vi "InitActuators.vi"   [LabVIEW 2020]
doc: "This VI initializes miscellaneous devices such as the compressor and any decorations."
uses:
  <vilib>/Rock Robotics/WPI/Utilities/WPI_GetSetVariantRefNum.vi
  <vilib>/Rock Robotics/WPI/ThirdParty/Phoenix-LabVIEW/Motor Controller/Controls/CTRE_Phoenix_MotorControl_TalonFXInvertType.ctl
  <vilib>/Rock Robotics/WPI/ThirdParty/Phoenix-LabVIEW/Motor Controller/Controls/CTRE_Phoenix_MotorControl_NeutralMode.ctl
  <vilib>/Rock Robotics/WPI/ThirdParty/Phoenix-LabVIEW/Motor Controller/Controls/CTRE_Phoenix_MotorControl_FeedbackDevice_TalonFX.ctl
  <vilib>/Rock Robotics/WPI/ThirdParty/Phoenix-LabVIEW/Motor Controller/Controls/CTRE_Phoenix_MotorControl_SupplyCurrentLimitConfiguration.ctl
  <vilib>/Rock Robotics/WPI/ThirdParty/Phoenix-LabVIEW/Motor Controller/Controls/CTRE_Phoenix_MotorControl_StatusFrameEnhanced.ctl
  GlobalActuators.vi
types:
  T1 = typedef "CTRE_Phoenix_MotorControl_StatusFrameEnhanced.ctl" = u16
  T2 = typedef "CTRE_Phoenix_MotorControl_SupplyCurrentLimitConfiguration.ctl" = cluster{"Enable?":bool, "Current Limit":dbl, "Threshold Current":dbl, "Threshold Time":dbl}
  T3 = typedef "CTRE_Phoenix_MotorControl_FeedbackDevice_TalonFX.ctl" = i8
  T4 = typedef "CTRE_Phoenix_MotorControl_NeutralMode.ctl" = enum8{"EEPROMSetting", "Override to Coast", "Override to Brake"}
  T5 = typedef "CTRE_Phoenix_MotorControl_TalonFXInvertType.ctl" = enum16{"Counter-Clockwise", "Clockwise"}
  T6 = typedef "WPI_MotorControlDeviceRef.ctl" = cluster{"DeviceStatus":errorcluster, "Type":T7, "PWM":cluster{"PWM Channel":T8, "DeadBand":T9}, "CAN":cluster{"Device Number":u8, "SetOutput VI Ref":variant, "GetOutput VI Ref":variant, "Enable VI Ref":variant, "Disable VI Ref":variant, "Data":variant}, "Invert":bool, "DIO PWM":cluster{"PWM \"Enable\" Channel":T8, "DIOChannel":T10, "PWM Rate":dbl}}
  T7 = typedef "WPI_MotorControlType.ctl" = enum16{"PWM", "CAN", "DIO PWM"}
  T8 = typedef "FPGA_DIOPWMChannel.ctl" = enum8{"PWM 0", "PWM 1", "PWM 2", "PWM 3", "PWM 4", "PWM 5", "PWM 6", "PWM 7", "PWM 8", "PWM 9", "PWM MXP 0", "PWM MXP 1", "PWM MXP 2", "PWM MXP 3", "PWM MXP 4", "PWM MXP 5", "PWM MXP 6", "PWM MXP 7", "PWM MXP 8", "PWM MXP 9", "Invalid"}
  T9 = typedef "WPI_PWMDeadband.ctl" = cluster{"Name":string, "maxPositivePwm":i32, "minPositivePwm":i32, "centerPwm":i32, "maxNegativePwm":i32, "minNegativePwm":i32, "angularRange":u16}
  T10 = typedef "FPGA_DIOChannel.ctl" = enum8{"DIO 0", "DIO 1", "DIO 2", "DIO 3", "DIO 4", "DIO 5", "DIO 6", "DIO 7", "DIO 8", "DIO 9", "DIO MXP 0", "DIO MXP 1", "DIO MXP 2", "DIO MXP 3", "DIO MXP 4", "DIO MXP 5", "DIO MXP 6", "DIO MXP 7", "DIO MXP 8", "DIO MXP 9", "DIO MXP 10", "DIO MXP 11", "DIO MXP 12", "DIO MXP 13", "DIO MXP 14", "DIO MXP 15", "SPI Port CS1", "SPI Port CS2", "SPI Port CS3", "SPI Port MISO", "SPI Port MOSI", "Invalid"}
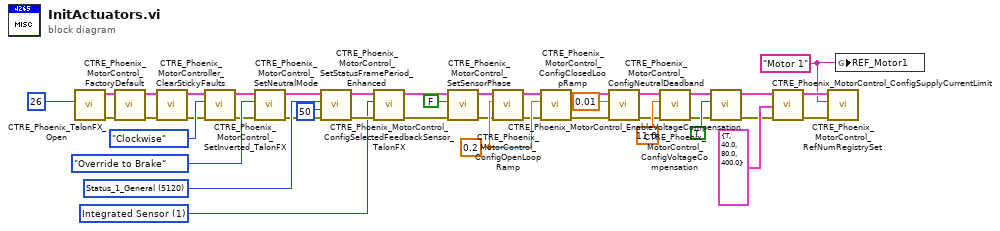
[diagram p0: block diagram]
diagram:
  w25 = T1 5120 items=["Status_1_General"=5120, "Status_2_Feedback0"=5184, "Status_3_Quadrature"=5248, "Status_4_AinTempVbat"=5312, "Status_6_Misc"=5440, "Status_7_CommStatus"=5504, "Status_8_PulseWidth"=5568, "Status_9_MotProfBuffer"=5632, "Status_10_MotionMagic"=5696, "Status_11_UartGadgeteer"=5760, "Status_12_Feedback1"=5824, "Status_13_Base_PIDF0"=5888, "Status_14_Turn_PIDF1"=5952, "Status_15_FirmwareApiStatus"=6016, "Status_Brushless_Current"=4672] ("Status Frame")
  w1 = "Motor 1" ("refnum name")
  w29 = 0.2 ("secondsFromNeutralToFull")
  w4 = T3 1 items=["Integrated Sensor"=1, "Sensor Sum (S0 + S1)"=9, "Sensor Difference (D0 - D1)"=10, "Remote Source 0"=11, "Remote Source 1"=12, "None"=14, "Software Emulated"=15] ("Talon FX Feedback Device")
  n1 = call <vilib>:"CTRE_Phoenix_TalonFX_Open.vi"("Device Number"=u8 26) -> ("error out"=w18:errorcluster, "PhoenixMotorControlDevRef"=w34:T6)  [unwired: 9 in]
  n2 = call <vilib>:"CTRE_Phoenix_MotorControl_FactoryDefault.vi"("error in"=w18, "PhoenixMotorControlDevRef"=w34) -> ("error out"=w19:errorcluster, "PhoenixMotorControlDevRef"=w35:T6)  [unwired: 8 in]
  n3 = call <vilib>:"CTRE_Phoenix_MotorController_ClearStickyFaults.vi"("error in"=w19, "PhoenixMotorControlDevRef"=w35) -> ("error out"=w20:errorcluster, "PhoenixMotorControlDevRef"=w36:T6)  [unwired: 8 in]
  n4 = call <vilib>:"CTRE_Phoenix_MotorControl_SetInverted_TalonFX.vi"("error in (no error)"=w20, "Invert Type"=CTRE_Phoenix_MotorControl_TalonFXInvertType."Clockwise", "PhoenixMotorControlDevRef"=w36) -> ("error out"=w21:errorcluster, "PhoenixMotorControlDevRef"=w37:T6)  [unwired: 7 in]
  n5 = call <vilib>:"CTRE_Phoenix_MotorControl_SetNeutralMode.vi"("error in (no error)"=w21, "Motor Control Neutral Mode"=CTRE_Phoenix_MotorControl_NeutralMode."Override to Brake", "PhoenixMotorControlDevRef"=w37) -> ("error out"=w22:errorcluster, "PhoenixMotorControlDevRef"=w41:T6)  [unwired: 7 in]
  n6 = call <vilib>:"CTRE_Phoenix_MotorControl_SetStatusFramePeriod_Enhanced.vi"("error in (no error)"=w22, "periodMs"=50, "Status Frame"=w25, "PhoenixMotorControlDevRef"=w41) -> ("error out"=w23:errorcluster, "PhoenixMotorControlDevRef"=w24:T6)  [unwired: 6 in]
  n7 = call <vilib>:"CTRE_Phoenix_MotorControl_ConfigSelectedFeedbackSensor_TalonFX.vi"("error in (no error)"=w23, "Talon FX Feedback Device"=w4, "PhoenixMotorControlDevRef"=w24) -> ("error out"=w12:errorcluster, "PhoenixMotorControlDevRef"=w14:T6)  [unwired: 7 in]
  n8 = call <vilib>:"CTRE_Phoenix_MotorControl_SetSensorPhase.vi"("error in (no error)"=w12, "PhaseSensor"=FALSE, "PhoenixMotorControlDevRef"=w14) -> ("error out"=w11:errorcluster, "PhoenixMotorControlDevRef"=w13:T6)  [unwired: 7 in]
  n9 = call <vilib>:"CTRE_Phoenix_MotorControl_ConfigOpenLoopRamp.vi"("error in (no error)"=w11, "secondsFromNeutralToFull"=w29, "PhoenixMotorControlDevRef"=w13) -> ("error out"=w17:errorcluster, "PhoenixMotorControlDevRef"=w38:T6)  [unwired: 7 in]
  n10 = call <vilib>:"CTRE_Phoenix_MotorControl_ConfigClosedLoopRamp.vi"("error in (no error)"=w17, "secondsFromNeutralToFull"=w29, "PhoenixMotorControlDevRef"=w38) -> ("error out"=w8:errorcluster, "PhoenixMotorControlDevRef"=w9:T6)  [unwired: 7 in]
  n11 = call <vilib>:"CTRE_Phoenix_MotorControl_ConfigNeutralDeadband.vi"("error in (no error)"=w8, "Percent Deadband"=0.01, "PhoenixMotorControlDevRef"=w9) -> ("error out"=w7:errorcluster, "PhoenixMotorControlDevRef"=w6:T6)  [unwired: 7 in]
  n12 = call <vilib>:"CTRE_Phoenix_MotorControl_ConfigVoltageCompensation.vi"("error in (no error)"=w7, "Saturation Voltage"=11.0, "PhoenixMotorControlDevRef"=w6) -> ("error out"=w16:errorcluster, "PhoenixMotorControlDevRef"=w39:T6)  [unwired: 7 in]
  n13 = call <vilib>:"CTRE_Phoenix_MotorControl_EnableVoltageCompensation.vi"("error in (no error)"=w16, "Enable Voltage Compensation?"=TRUE, "PhoenixMotorControlDevRef"=w39) -> ("error out"=w15:errorcluster, "PhoenixMotorControlDevRef"=w40:T6)  [unwired: 7 in]
  n14 = call <vilib>:"CTRE_Phoenix_MotorControl_ConfigSupplyCurrentLimit.vi"("error in (no error)"=w15, "Supply Current Limit Configuration"=T2 {"Enable?"=TRUE, "Current Limit"=40.0, "Threshold Current"=80.0, "Threshold Time"=400.0}, "PhoenixMotorControlDevRef"=w40) -> ("error out"=w2:errorcluster, "PhoenixMotorControlDevRef"=w3:T6)  [unwired: 7 in]
  n15 = call <vilib>:"CTRE_Phoenix_MotorControl_RefNumRegistrySet.vi"("error in (no error)"=w2, "refnum name"=w1, "PhoenixMotorControlDevRef"=w3) -> ()  [unwired: 7 in, 2 out]
  n16 = global write "GlobalActuators.vi" "REF_Motor1"(w1) -> ()
